vi "Sampler.vi"(8 "error in (no error)":errorcluster, 10 "Signal List":string(combo), 11 "Sampler":refnum<k24>) -> (0 "error out":errorcluster, 2 "Signal Value":dbl, 3 "GetSignals":string[](array[string]))   [LabVIEW 2011]
doc: "Shows the signals from the sampler."
uses:
  C:/Program Files/Metrohm Autolab/Autolab SDK 1.10/EcoChemie.Autolab.Sdk.dll
  EcoChemie.Autolab.Sdk.dll
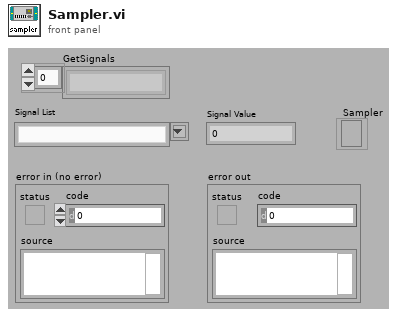
[diagram p1: front panel]
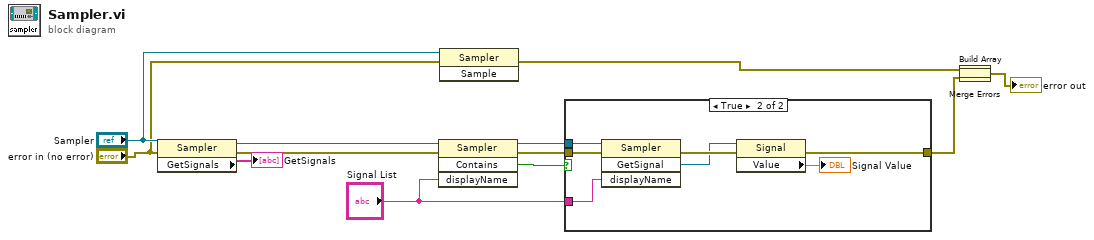
[diagram p0: block diagram]
diagram:
  n1 = property class="Sampler"(reference="Sampler", error in="error in (no error)") -> (reference out=w11:refnum<k24>, error out=w10:errorcluster, "GetSignals"=→"GetSignals":string[])
  n2 = invoke class="Sampler" method="Contains"(reference=w11, error in=w10, "displayName"="Signal List") -> (reference out=w8:refnum<k24>, error out=w12:errorcluster, "Contains"=w13:bool)  [unwired: 1 in, 1 out]
  n3 = invoke class="Sampler" method="Sample"(reference="Sampler", error in="error in (no error)") -> (error out=w4:errorcluster)  [unwired: 1 in, 2 out]
  n4 = case shown="True" w13 {
    tunnel: [w14 w20] -> w3
    tunnel: w12 -> [w14 w19]
    tunnel: "Signal List" -> [_ w16]
    tunnel: w8 -> [_ w15]
    frame False {
    }
    frame True {
      n5 = invoke class="Sampler" method="GetSignal"(reference=w15, error in=w19, "displayName"=w16) -> (error out=w18:errorcluster, "GetSignal"=w17:refnum<k24>)  [unwired: 1 in, 2 out]
      n6 = property class="Signal"(reference=w17, error in=w18) -> (error out=w20:errorcluster, "Value"=→"Signal Value":dbl)  [unwired: 1 out]
    }
  }
  n7 = Build Array(w4, w3) -> (w1:errorcluster[])
  n8 = Merge Errors(w1) -> (→"error out":errorcluster)
